vi "ExecuteButtonAction.vi"(8 "Error In":errorcluster, 9 "WaitForReply":bool, 10 "Command":string, 11 "reference in":refnum<class "UserManager.lvclass">) -> (0 "Error Out":errorcluster, 3 "reference in":refnum<class "UserManager.lvclass">)   [LabVIEW 2021, in "UserMananger.lvlib" / "UserManager.lvclass"]
uses:
  UserManager.lvclass
  C:/Localdata/Projects/TriekselSoft/TriekselsoftApplicationFramework/Source/.Externals/Library_TAF_ApplicationFramework/TAFBaseGUI/TAFBaseGUI.lvclass
  Library_TAF_ApplicationFramework/TAFBaseGUI/TAFBaseGUI.lvclass
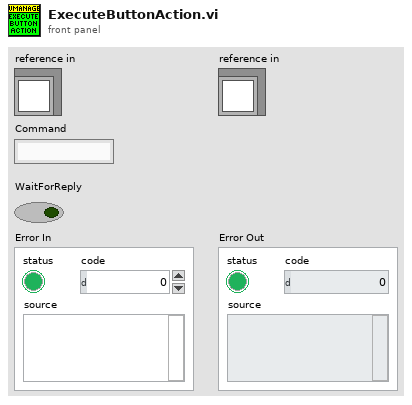
[diagram p1: front panel]
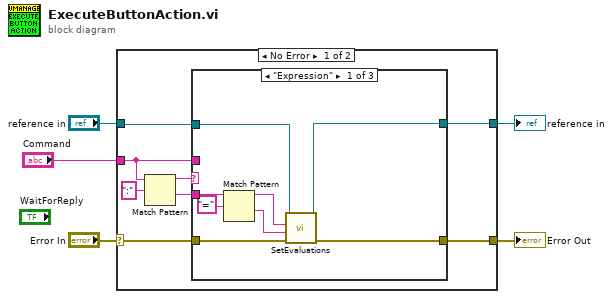
[diagram p0: block diagram]
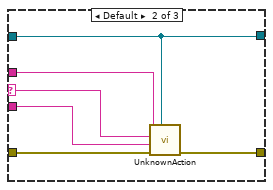
[diagram p2: hidden frame]
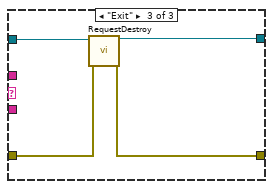
[diagram p3: hidden frame]
diagram:
  n1 = case shown="No Error" "Error In" {
    selector: "Error In" -> [w8 w33]
    tunnel: [w7 w33] -> w4
    tunnel: [w12 w32] -> w2
    tunnel: "reference in" -> [w13 w32]
    tunnel: "Command" -> [w6 _]
    frame No Error {
      n2 = Match Pattern(string=w6, regular expression=":") -> (before substring=w11:string, after substring=w9:string)  [unwired: 1 in, 2 out]
      n3 = case shown="\"Expression\"" w11 {
        selector: w11 -> [_ w24 _]
        tunnel: w13 -> [w17 w22 w31]
        tunnel: [w16 w22 w30] -> w12
        tunnel: w9 -> [w21 w23 _]
        tunnel: [w18 w27 w28] -> w7
        tunnel: w8 -> [w19 w26 w29]
        tunnel: w6 -> [_ w25 _]
        frame "Expression" {
          n4 = Match Pattern(string=w21, regular expression="=") -> (before substring=w15:string, after substring=w14:string)  [unwired: 1 in, 2 out]
          n5 = call-dynamic "SetEvaluations.vi"("Error In"=w19, "Value"=w14, "Label"=w15, "reference in"=w17) -> ("Error Out"=w18:errorcluster, "reference in"=w16:refnum<class "UserManager.lvclass">)  [unwired: 6 in]
        }
        frame Default {
          n6 = call "UnknownAction.vi"("Object"=w22, "error in (no error)"=w26, "Parameters"=w23, "SubCommand"=w24, "FullCommand"=w25) -> ("error out"=w27:errorcluster)  [unwired: 6 in]
        }
        frame "Exit" {
          n7 = call "RequestDestroy.vi"("Error In"=w29, "reference in"=w31) -> ("Error Out"=w28:errorcluster, "reference out"=w30:refnum<class "UserManager.lvclass">)  [unwired: 8 in]
        }
      }
    }
    frame Error {
    }
  }
  "Error Out" <- w4
  "reference in" <- w2
